vi "MSP430 Simple Debugger.vi"() -> ()   [LabVIEW 2014]
uses:
  <vilib>/regexp/Match Regular Expression.xnode
panel:
  in  "STOP DEBUG":bool
  in  "button DISCONNECT":bool
  in  "button CONNECT":bool
  in  "button halt":bool
  in  "button RUN":bool
  in  "button breakpoint":bool
  in  "breakpoint line num.":i32=42
  in  "error in":errorcluster
  out "result string":string
  out "error out":errorcluster
  out "Errors":string
  out "Command Return Value(s)":string
  in  "input file (.out)":path=path "C:/Users/Simon Gurfunkel/Documents/LabVIEW_projects/LabVIEW-Universal-Transcriptor/Transcriptors/2/Examples - Arduino/Example_MSP430_Blink/blink.out"
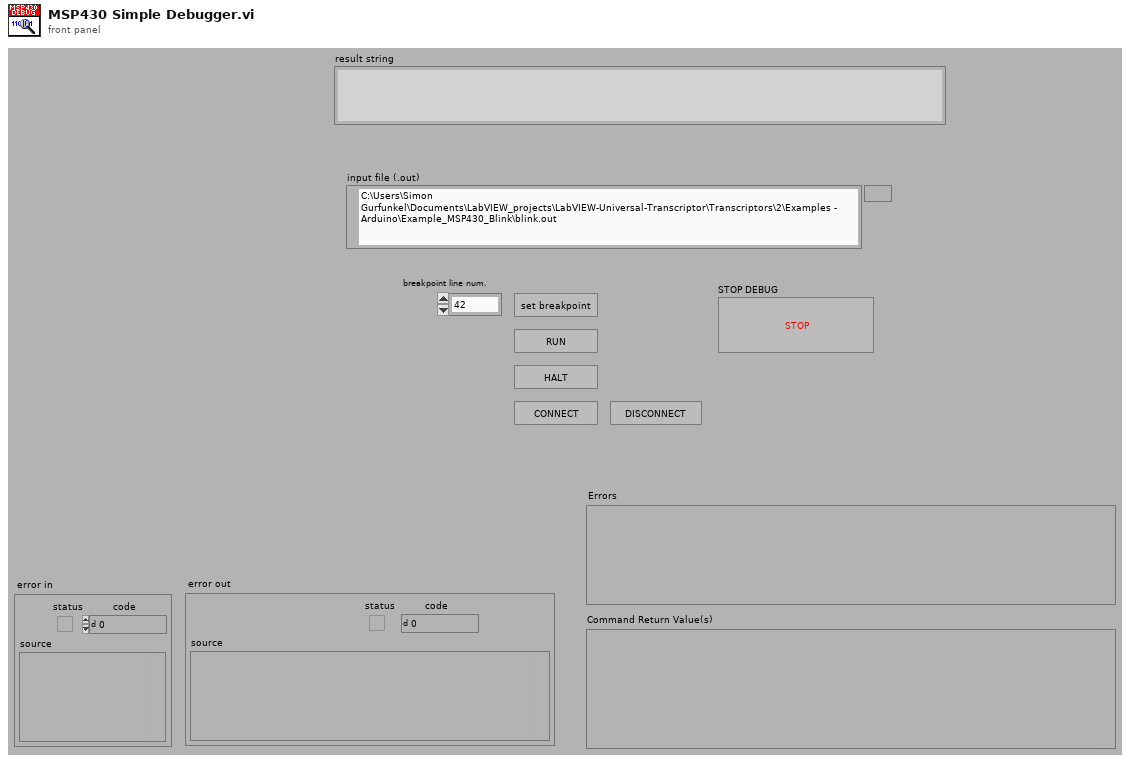
[diagram p1: front panel]
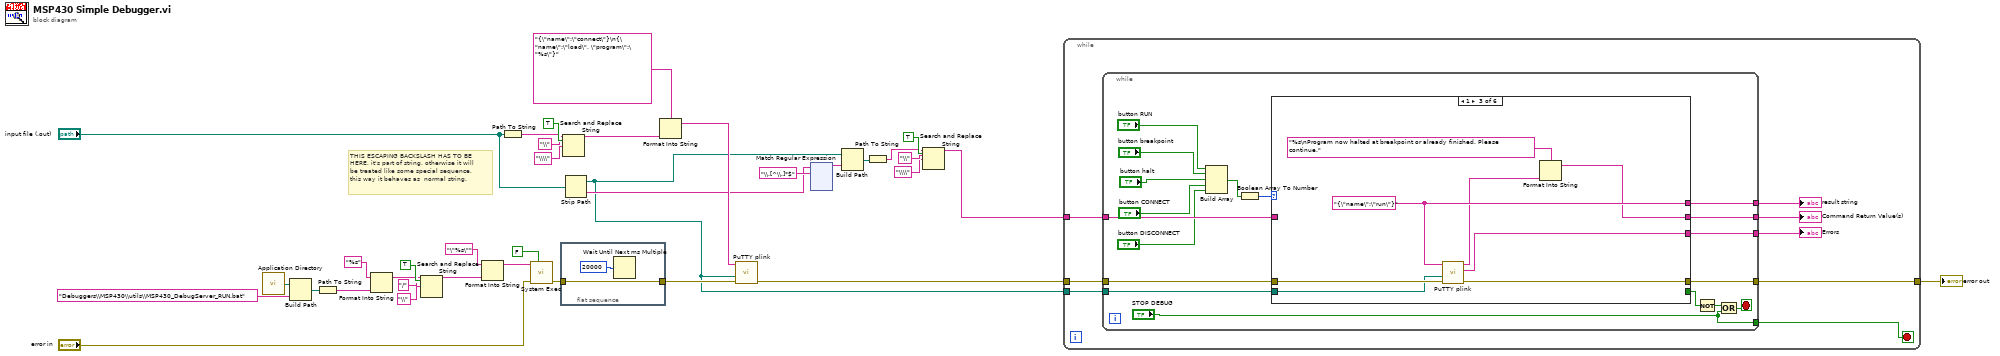
[diagram p0: block diagram]
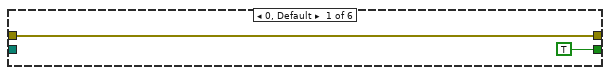
[diagram p2: hidden frame]
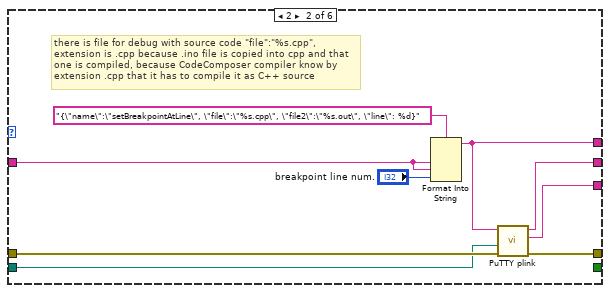
[diagram p3: hidden frame]
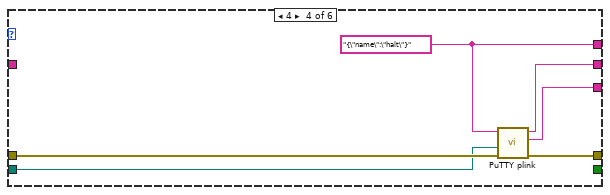
[diagram p4: hidden frame]
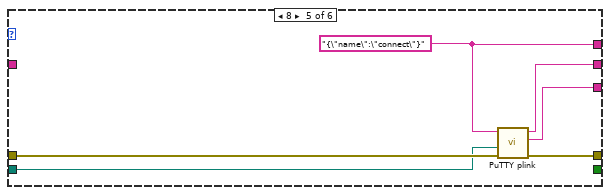
[diagram p5: hidden frame]
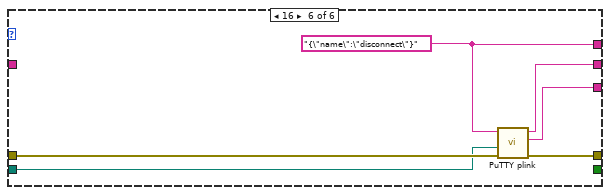
[diagram p6: hidden frame]
diagram:
  # "THIS ESCAPING BACKSLASH HAS TO BE HERE, it's part of string, otherwise it will be treated like some special sequence, this way it behaves as  normal string."
  n1 = call <vilib>:"Application Directory.vi"() -> ("Application Directory"=w34:path)
  n2 = Build Path(base path=w34, name or relative path="Debuggers\\MSP430\\utils\\MSP430_DebugServer_RUN.bat" ("standard input")) -> (appended path=w32:path)
  n3 = Path To String(path=w32) -> (string=w28:string)
  n4 = Format Into String(format string="%s", w28) -> (resulting string=w23:string)  [unwired: 2 in, 1 out]
  n5 = Search and Replace String(replace all?=TRUE ("replace all? (F)"), input string=w23, search string="/", replace string="\\" ("search string")) -> (result string=w22:string)  [unwired: 4 in, 3 out]
  n6 = Format Into String(format string="\"%s\"", w22) -> (resulting string=w20:string)  [unwired: 2 in, 1 out]
  n7 = Path To String(path="input file (.out)") -> (string=w14:string)
  n8 = call <vilib>:"System Exec.vi"("wait until completion? (T)"=FALSE, "error in (no error)"="error in", "command line"=w20) -> ("error out"=w35:errorcluster)  [unwired: 3 in, 5 out]
  n9 = flat-sequence {
    tunnel: [w37] -> w29
    tunnel: w35 -> [w37]
    frame #0 {
      n10 = Wait Until Next ms Multiple(millisecond multiple=u32 20000) -> ()  [unwired: 1 out]
    }
  }
  n11 = Search and Replace String(replace all?=TRUE ("replace all? (F)"), input string=w14, search string="\\", replace string="\\\\" ("search string")) -> (result string=w13:string)  [unwired: 4 in, 3 out]
  n12 = Strip Path(path="input file (.out)") -> (stripped path=w7:path, name=w9:string)
  n13 = Format Into String(format string="{\"name\":\"connect\"}\n{\"name\":\"load\", \"program\":\"%s\"}", w13) -> (resulting string=w30:string)  [unwired: 2 in, 1 out]
  n14 = call "PuTTY plink.vi"("error in"=w29, "working directory"=w7, "Command(s) to Execute"=w30) -> ("error out"=w12:errorcluster)  [unwired: 6 in, 2 out]
  n15 = xnode ("Match Regular Expression")("input string"=w9, "regular expression"="\\.[^\\.]*$" ("input string")) -> ("before match"=w8:string)  [unwired: 4 in, 4 out]
  n16 = Build Path(base path=w7, name or relative path=w8) -> (appended path=w3:path)
  n17 = Path To String(path=w3) -> (string=w2:string)
  n18 = Search and Replace String(replace all?=TRUE ("replace all? (F)"), input string=w2, search string="\\", replace string="\\\\" ("search string")) -> (result string=w1:string)  [unwired: 4 in, 3 out]
  n19 = while {
    tunnel: w7 -> [w44]
    tunnel: w1 -> [w43]
    tunnel: w12 -> [w46]
    tunnel: [w45] -> w11
    stop <- w39 stop-if-true
    n20 = while {
      tunnel: w44 -> [w62]
      tunnel: [w59] -> w41
      tunnel: [w58] -> w40
      tunnel: w46 -> [w64]
      tunnel: [w63] -> w45
      tunnel: w43 -> [w61]
      tunnel: [w60] -> w42
      tunnel: ["STOP DEBUG"] -> w39
      stop <- w48 stop-if-true
      n21 = Build Array("button RUN", "button breakpoint", "button halt", "button CONNECT", "button DISCONNECT") -> (w51:bool[])
      n22 = Boolean Array To Number(Boolean array=w51) -> (number=w57:u32)
      n23 = case shown="1" w57 {
        tunnel: w64 -> [w66 w74 w83 w89 w95 w101]
        tunnel: [w66 w73 w82 w88 w94 w100] -> w63
        tunnel: w62 -> [_ w71 w81 w87 w93 w99]
        tunnel: w61 -> [_ w70 _ _ _ _]
        tunnel: [_ w69 w76 w86 w92 w98] -> w60
        tunnel: [_ w68 w80 w85 w91 w97] -> w59
        tunnel: [_ w67 w79 w84 w90 w96] -> w58
        tunnel: [TRUE _ _ _ _ _] -> w50
        frame 0, Default {
        }
        frame 2 {
          # "there is file for debug with source code \"file\":\"%s.cpp\", extension is .cpp because .ino file is copied into cpp and that one is compiled, because CodeComposer compiler know by extension .cpp that it has to compile it as C++ source"
          n24 = Format Into String(format string="{\"name\":\"setBreakpointAtLine\", \"file\":\"%s.cpp\", \"file2\":\"%s.out\", \"line\": %d}", w70, w70, "breakpoint line num.") -> (resulting string=w67:string)  [unwired: 2 in, 1 out]
          n25 = call "PuTTY plink.vi"("error in"=w74, "working directory"=w71, "Command(s) to Execute"=w67) -> ("error out"=w73:errorcluster, "Errors"=w68:string, "Command Return Value(s)"=w69:string)  [unwired: 6 in]
        }
        frame 1 {
          w79 = "{\"name\":\"run\"}" ("format string")
          n26 = call "PuTTY plink.vi"("error in"=w83, "working directory"=w81, "Command(s) to Execute"=w79) -> ("error out"=w82:errorcluster, "Errors"=w80:string, "Command Return Value(s)"=w77:string)  [unwired: 6 in]
          n27 = Format Into String(format string="%s\nProgram now halted at breakpoint or already finished. Please continue.", w77) -> (resulting string=w76:string)  [unwired: 2 in, 1 out]
        }
        frame 4 {
          w84 = "{\"name\":\"halt\"}" ("format string")
          n28 = call "PuTTY plink.vi"("error in"=w89, "working directory"=w87, "Command(s) to Execute"=w84) -> ("error out"=w88:errorcluster, "Errors"=w85:string, "Command Return Value(s)"=w86:string)  [unwired: 6 in]
        }
        frame 8 {
          w90 = "{\"name\":\"connect\"}" ("format string")
          n29 = call "PuTTY plink.vi"("error in"=w95, "working directory"=w93, "Command(s) to Execute"=w90) -> ("error out"=w94:errorcluster, "Errors"=w91:string, "Command Return Value(s)"=w92:string)  [unwired: 6 in]
        }
        frame 16 {
          w96 = "{\"name\":\"disconnect\"}" ("format string")
          n30 = call "PuTTY plink.vi"("error in"=w101, "working directory"=w99, "Command(s) to Execute"=w96) -> ("error out"=w100:errorcluster, "Errors"=w97:string, "Command Return Value(s)"=w98:string)  [unwired: 6 in]
        }
      }
      n31 = Not(x=w50) -> (.not. x?=w49:bool)
      n32 = Or(x=w49, y="STOP DEBUG") -> (x .or. y?=w48:bool)
    }
    "Command Return Value(s)" <- w42
    "Errors" <- w41
    "result string" <- w40
  }
  "error out" <- w11
